vi "Colour_Sampling.vi"() -> (0 "Just the ascending angles":dbl[](array[numeric]), 2 "All colours in ascending angles: R/G/B/num/angle":dbl[][](array[numeric]))   [LabVIEW 2017]
uses:
  ec4b2f25-54d4-4e98-8021-b3fe3c98dd16.vi
  <vilib>/Array/Sort 2D Array - Pop Stack.vi
  <vilib>/Array/Sort 2D Array - Push Stack.vi
panel:
  out "RGB/4/angles for black":dbl[][](array[numeric])
  out "RGB/3/angles for yellow":dbl[][](array[numeric])
  out "RGB/2/angles for green":dbl[][](array[numeric])
  out "RGB/1/angles for red":dbl[][](array[numeric])
  in  "Stop black":bool
  out "Loops for black":i32
  out "Black array":u8[][](array[numeric])
  out "Black angle array":dbl[](array[numeric])
  in  "A/12C 2":tag="B/I2C"
  in  "Start black":bool
  out "Yellow angle array":dbl[](array[numeric])
  out "Yellow array":u8[][](array[numeric])
  out "Green angle array":dbl[](array[numeric])
  out "Green array":u8[][](array[numeric])
  out "Red angle array":dbl[](array[numeric])
  out "Red array":u8[][](array[numeric])
  out "Loops for yellow":i32
  in  "Stop yellow":bool
  in  "Start yellow":bool
  in  "A/12C":tag="B/I2C"
  in  "Stop green":bool
  out "Loops for green":i32
  in  "Start green":bool
  in  "A/12C":tag="B/I2C"
  in  "Start red":bool
  in  "A/12C":tag="B/I2C"
  in  "Stop red":bool
  out "Loops for red":i32
  # "1. START\n2. STOP\n3. DO IT"
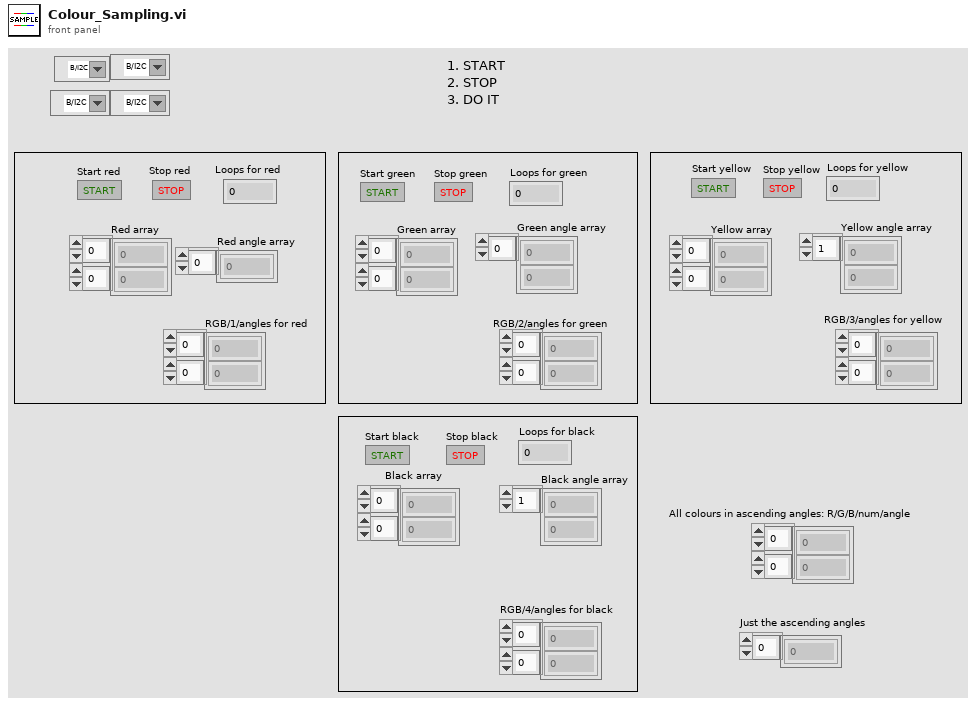
[diagram p1: front panel]
types:
  T1 = typedef "I2C.lvlib/I2C Reference.ctl" = cluster{"myRIO Reference":T2, "I2C Channels Enum":T6, "I2C Configuration":T7}
  T2 = typedef "myRIO Generic Hardware Reference.ctl" = cluster{"myRIO Model":T3, "myRIO Hardware Reference":T4}
  T3 = typedef "Hardware Version Enum.ctl" = enum16{"Unknown", "myRIO-1900", "myRIO-1950", "roboRIO", "NI ELVIS RIO CM"}
  T4 = typedef "myRIO v1.0 Reference.ctl" = cluster{"Generic FPGA Reference":T5, "Allow multiple opens":bool}
  T5 = typedef "Generic FPGA Reference.ctl" = refnum<k20>
  T6 = typedef "I2C Channels Enum.ctl" = enum16{"Not Connected", "A/I2C", "B/I2C", "I2C/I2C"}
  T7 = typedef "I2C.lvlib/I2C Configuration.ctl" = cluster{"I2C Transfer Rate":T8}
  T8 = typedef "I2C.lvlib/I2C Transfer Rate.ctl" = enum16{"Standard mode (100 kbps)", "Fast mode (400 kbps)"}
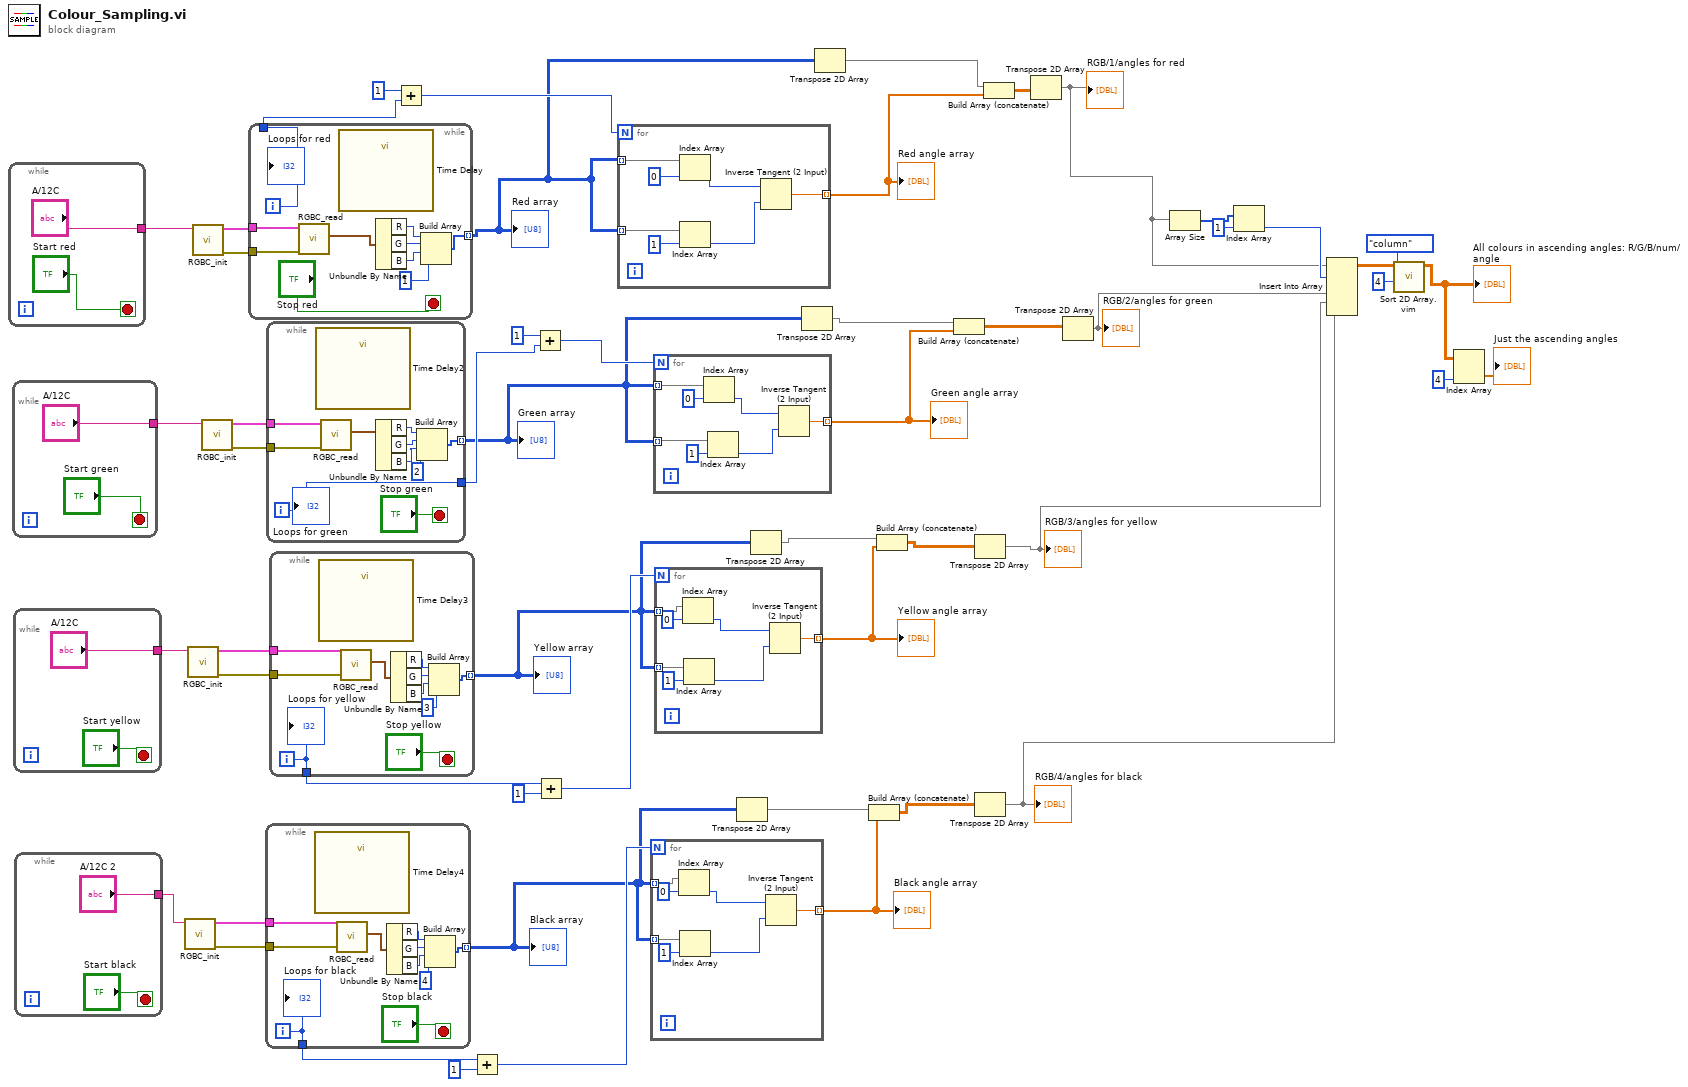
[diagram p0: block diagram]
diagram:
  n1 = while {
    tunnel: ["A/12C"] -> w52
    stop <- "Start red" stop-if-true
  }
  n2 = while {
    tunnel: ["A/12C"] -> w50
    stop <- "Start green" stop-if-true
  }
  n3 = while {
    tunnel: ["A/12C"] -> w47
    stop <- "Start yellow" stop-if-true
  }
  n4 = while {
    tunnel: ["A/12C 2"] -> w44
    stop <- "Start black" stop-if-true
  }
  n5 = call "RGBC_init.vi"("Channel Name"=w44) -> ("error out"=w42:errorcluster, "I2C Ref Out"=w43:T1)  [unwired: 9 in]
  n6 = call "RGBC_init.vi"("Channel Name"=w47) -> ("error out"=w45:errorcluster, "I2C Ref Out"=w46:T1)  [unwired: 9 in]
  n7 = call "RGBC_init.vi"("Channel Name"=w52) -> ("error out"=w53:errorcluster, "I2C Ref Out"=w51:T1)  [unwired: 9 in]
  n8 = call "RGBC_init.vi"("Channel Name"=w50) -> ("error out"=w48:errorcluster, "I2C Ref Out"=w49:T1)  [unwired: 9 in]
  n9 = while {
    tunnel: w53 -> [w71]
    tunnel: w51 -> [w70]
    tunnel: [w63] -> w28 mode=indexing
    tunnel: [w68] -> w41
    i -> [w68]
    stop <- "Stop red" stop-if-true
    n10 = call "RGBC_read.vi"("error in (no error)"=w71, "I2C Ref In"=w70) -> ("RGB"=w67:cluster{"R":u8, "G":u8, "B":u8})  [unwired: 7 in, 2 out]
    n11 = call "Time Delay"() -> ()  [unwired: 11 in, 1 out]
    n12 = Unbundle By Name(w67) -> ("R"=w66:u8, "G"=w65:u8, "B"=w64:u8)
    n13 = Build Array(w66, w65, w64, u8 1 ("element")) -> (w63:u8[])
    "Loops for red" <- w68
  }
  "Red array" <- w28
  n14 = while {
    tunnel: w43 -> [w81]
    tunnel: w42 -> [w80]
    tunnel: [w74] -> w17 mode=indexing
    tunnel: [w73] -> w34
    i -> [w73]
    stop <- "Stop black" stop-if-true
    n15 = call "Time Delay4"() -> ()  [unwired: 11 in, 1 out]
    n16 = call "RGBC_read.vi"("error in (no error)"=w80, "I2C Ref In"=w81) -> ("RGB"=w78:cluster{"R":u8, "G":u8, "B":u8})  [unwired: 7 in, 2 out]
    n17 = Unbundle By Name(w78) -> ("R"=w77:u8, "G"=w76:u8, "B"=w75:u8)
    n18 = Build Array(w77, w76, w75, u8 4 ("element")) -> (w74:u8[])
    "Loops for black" <- w73
  }
  "Black array" <- w17
  n19 = while {
    tunnel: w49 -> [w91]
    tunnel: w48 -> [w90]
    tunnel: [w84] -> w25 mode=indexing
    tunnel: [w83] -> w40
    i -> [w83]
    stop <- "Stop green" stop-if-true
    n20 = call "Time Delay2"() -> ()  [unwired: 11 in, 1 out]
    n21 = call "RGBC_read.vi"("error in (no error)"=w90, "I2C Ref In"=w91) -> ("RGB"=w88:cluster{"R":u8, "G":u8, "B":u8})  [unwired: 7 in, 2 out]
    n22 = Unbundle By Name(w88) -> ("R"=w86:u8, "G"=w87:u8, "B"=w85:u8)
    n23 = Build Array(w86, w87, w85, u8 2 ("element")) -> (w84:u8[])
    "Loops for green" <- w83
  }
  "Green array" <- w25
  n24 = while {
    tunnel: w46 -> [w101]
    tunnel: w45 -> [w100]
    tunnel: [w94] -> w21 mode=indexing
    tunnel: [w93] -> w37
    i -> [w93]
    stop <- "Stop yellow" stop-if-true
    n25 = call "Time Delay3"() -> ()  [unwired: 11 in, 1 out]
    n26 = call "RGBC_read.vi"("error in (no error)"=w100, "I2C Ref In"=w101) -> ("RGB"=w98:cluster{"R":u8, "G":u8, "B":u8})  [unwired: 7 in, 2 out]
    n27 = Unbundle By Name(w98) -> ("R"=w97:u8, "G"=w96:u8, "B"=w95:u8)
    n28 = Build Array(w97, w96, w95, u8 3 ("element")) -> (w94:u8[])
    "Loops for yellow" <- w93
  }
  "Yellow array" <- w21
  n29 = Add(x=1, y=w41) -> (x+y=w30:i32)
  n30 = Add(x=w34, y=1) -> (x+y=w33:i32)
  n31 = Add(x=1, y=w40) -> (x+y=w39:i32)
  n32 = Add(x=w37, y=1) -> (x+y=w36:i32)
  n33 = for {
    N: w30 -> [_]
    tunnel: w28 -> [w103] mode=indexing
    tunnel: w28 -> [w104] mode=indexing
    tunnel: [w108] -> w29 mode=indexing
    n34 = Index Array(array=w104, index=0) -> (element=w102:u8)
    n35 = Index Array(array=w103, index=1) -> (element=w105:u8)
    n36 = Inverse Tangent (2 Input)(1:w105, 2:w102) -> (0:w108:dbl)
  }
  "Red angle array" <- w29
  n37 = for {
    N: w33 -> [_]
    tunnel: w17 -> [w115] mode=indexing
    tunnel: w17 -> [w114] mode=indexing
    tunnel: [w109] -> w15 mode=indexing
    n38 = Index Array(array=w115, index=0) -> (element=w111:u8)
    n39 = Index Array(array=w114, index=1) -> (element=w110:u8)
    n40 = Inverse Tangent (2 Input)(1:w110, 2:w111) -> (0:w109:dbl)
  }
  "Black angle array" <- w15
  n41 = for {
    N: w39 -> [_]
    tunnel: w25 -> [w121] mode=indexing
    tunnel: [w116] -> w23 mode=indexing
    tunnel: w25 -> [_] mode=indexing
    n42 = Index Array(array=w121, index=0 ("index (row)")) -> (element=w118:u8)
    n43 = Index Array(array=w121, index=1 ("index (row)")) -> (element=w117:u8)
    n44 = Inverse Tangent (2 Input)(1:w117, 2:w118) -> (0:w116:dbl)
  }
  "Green angle array" <- w23
  n45 = for {
    N: w36 -> [_]
    tunnel: w21 -> [w128] mode=indexing
    tunnel: w21 -> [w127] mode=indexing
    tunnel: [w122] -> w19 mode=indexing
    n46 = Index Array(array=w128, index=0) -> (element=w124:u8)
    n47 = Index Array(array=w127, index=1) -> (element=w123:u8)
    n48 = Inverse Tangent (2 Input)(1:w123, 2:w124) -> (0:w122:dbl)
  }
  "Yellow angle array" <- w19
  n49 = Transpose 2D Array(2D array=w17) -> (transposed array=w16:u8[][])
  n50 = Transpose 2D Array(2D array=w21) -> (transposed array=w20:u8[][])
  n51 = Transpose 2D Array(2D array=w25) -> (transposed array=w24:u8[][])
  n52 = Transpose 2D Array(2D array=w28) -> (transposed array=w27:u8[][])
  n53 = Build Array (concatenate)(w16, w15) -> (w14:dbl[][])
  n54 = Build Array (concatenate)(w20, w19) -> (w18:dbl[][])
  n55 = Build Array (concatenate)(w24, w23) -> (w22:dbl[][])
  n56 = Transpose 2D Array(2D array=w18) -> (transposed array=w8:dbl[][])
  "RGB/3/angles for yellow" <- w8
  n57 = Transpose 2D Array(2D array=w14) -> (transposed array=w7:dbl[][])
  "RGB/4/angles for black" <- w7
  n58 = Build Array (concatenate)(w27, w29) -> (w26:dbl[][])
  n59 = Transpose 2D Array(2D array=w26) -> (transposed array=w10:dbl[][])
  "RGB/1/angles for red" <- w10
  n60 = Transpose 2D Array(2D array=w22) -> (transposed array=w9:dbl[][])
  "RGB/2/angles for green" <- w9
  n61 = Array Size(array=w10) -> (size(s)=w13:i32[])
  n62 = Index Array(array=w13, index=1) -> (element=w11:i32)
  n63 = Insert Into Array(array=w10, index (row)=w11, new element #1=w9, new element #2=w8, new element #3=w7) -> (w6:dbl[][])  [unwired: 1 in]
  n64 = call "Sort 2D Array.vim"("index"=4, "dimension to index (column)"=enum16{"column", "row"}."column", "2D array"=w6) -> ("sorted 2D array"=w3:dbl[][])  [unwired: 7 in, 1 out]
  "All colours in ascending angles: R/G/B/num/angle" <- w3
  n65 = Index Array(array=w3, index (col)=4 ("disabled index (col)")) -> (element=→"Just the ascending angles":dbl[])  [unwired: 1 in]
